vi "close_all.vi"(6 "Array of Controller Status":T1, 8 "error in (no error)":errorcluster, 9 "Hamamatsu_C9100-13.lvclass":refnum<class "Hamamatsu_C9100-13.lvclass">, 10 "HP83623A Generator Settings Array":T2, 11 "DDS Settings":T4={"Enable DDS"=TRUE, "Array of DDS Boxes"=[]} {"Array of DDS Boxes"."Array of DDS Channels (4)"."Channel Parameters"."Ref Clock Rate [kHz]" min=0.0}) -> (0 "error out":errorcluster)   [LabVIEW 2013, in "Experiment.lvclass"]
uses:
  Experiment/Experiment.lvclass
  DDS/DDS_Settings_Cluster.ctl
  DDS drivers v3/Array_of_DDS_Boxes.ctl
  DDS drivers v3/DDS_box_cluster.ctl
  DDS drivers v3/DDS_box_device_reference.ctl
  <vilib>/ni845x/ni845x.llb/ni845xControl.ctl
  DDS drivers v3/array_of_DDS_channels.ctl
  DDS drivers v3/DDS_channel.ctl
  DDS drivers v3/array_of_DDS_profiles.ctl
  DDS drivers v3/DDS_profile.ctl
  DDS drivers v3/DDS RAM mode.ctl
  GPIB/HP83623A_RF_Generator/HP83623A_array.ctl
  GPIB/HP83623A_RF_Generator/HP83623A.ctl
  Camera/Hamamatsu_C9100-13/Hamamatsu_C9100-13.lvclass
  PI_piezo/status.ctl
  GPIB/HP83623A_RF_Generator/HP83623A_RF_Generator.lvclass
  PI_piezo/PI_Piezo.lvclass
  DDS/DDS.lvclass
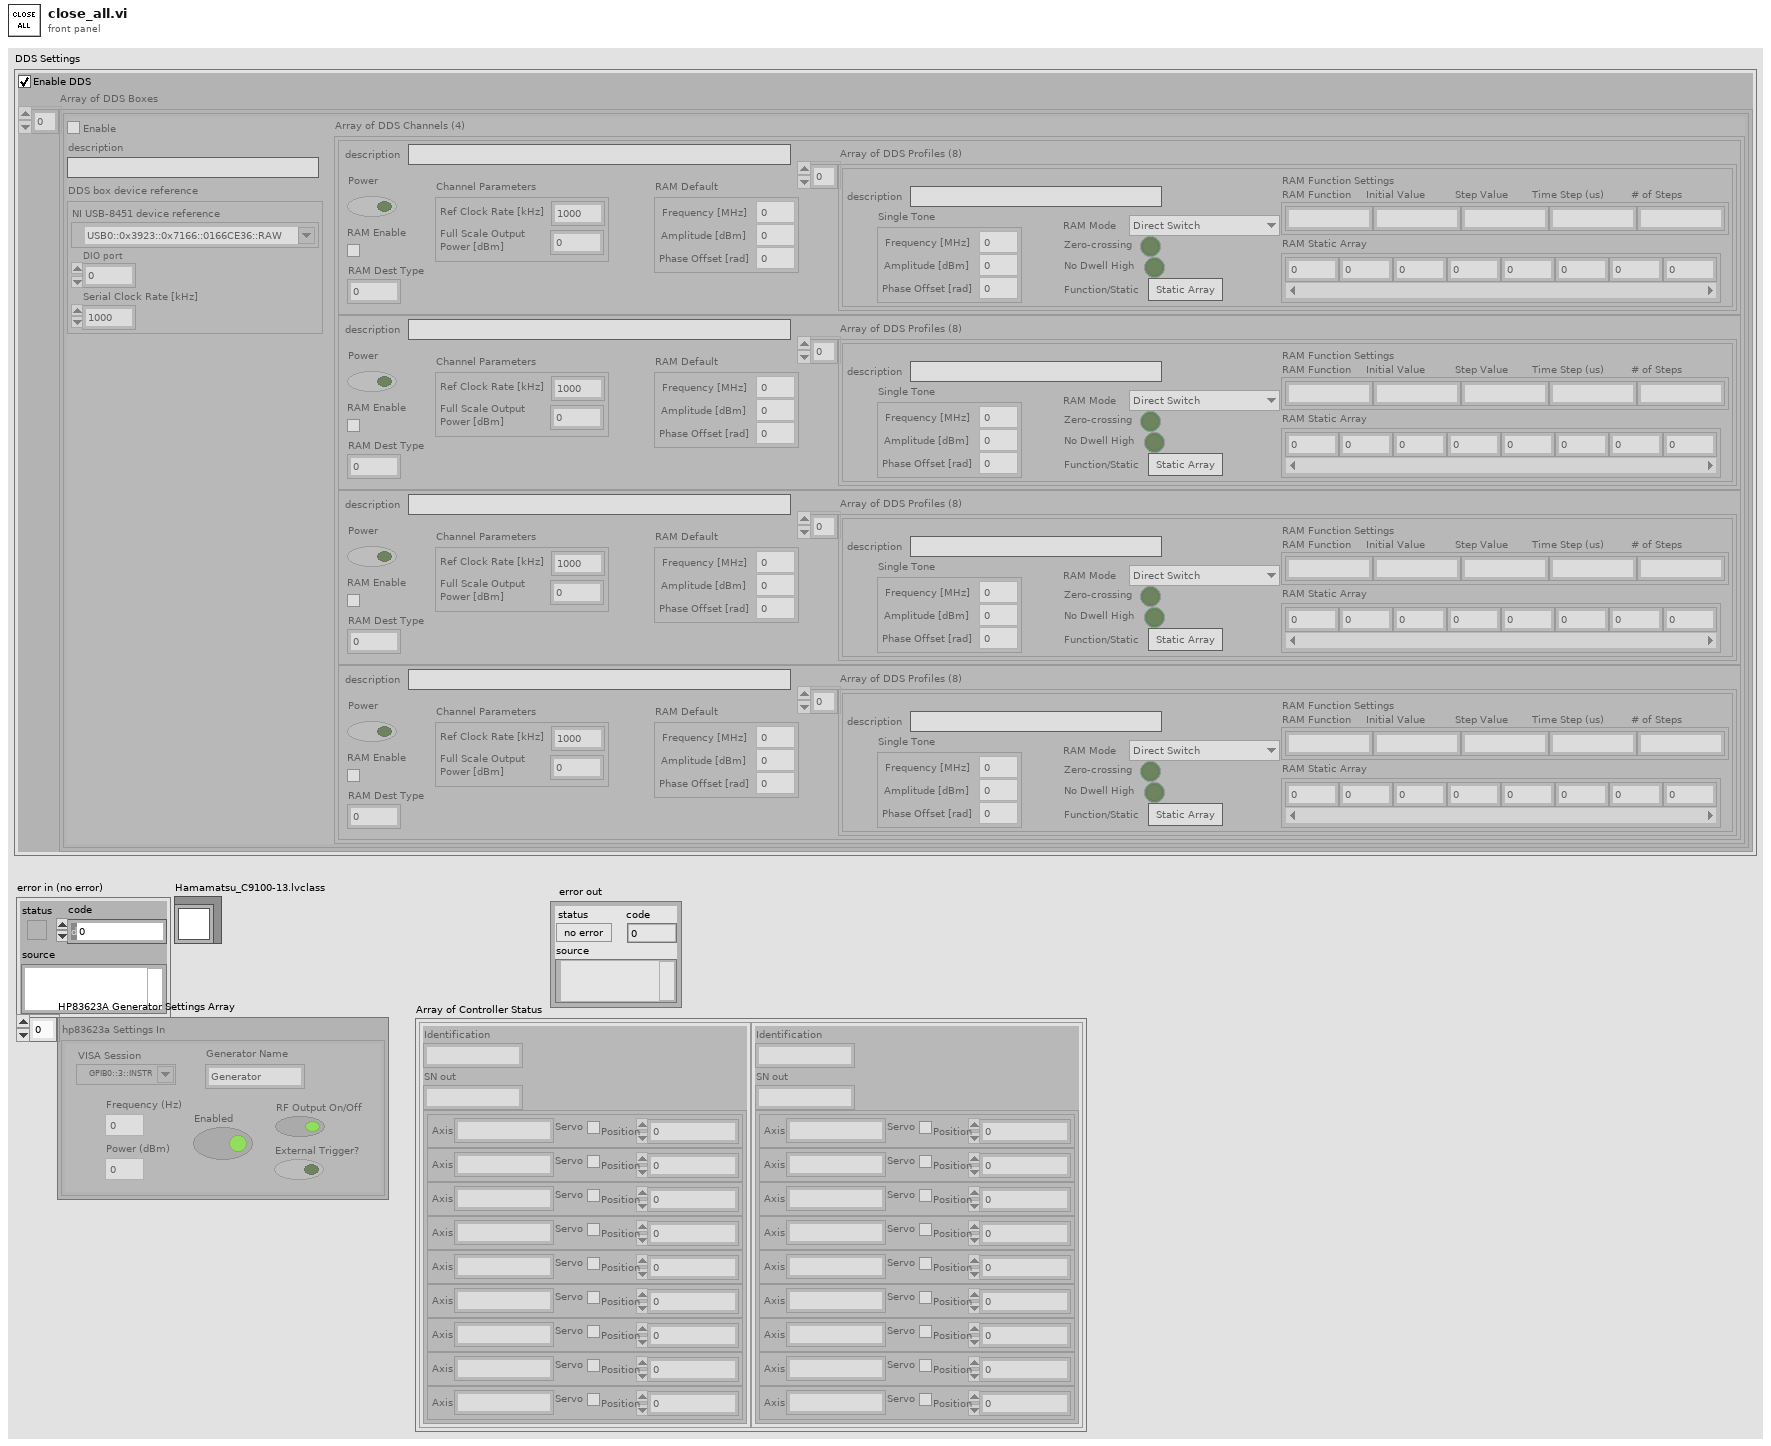
[diagram p1: front panel]
types:
  T1 = typedef "PI_Piezo.lvclass/status.ctl" = cluster{"Identification":string, "SN out":string, cluster{"Axis":string, "Servo":bool, "Position":dbl}[]}[]
  T2 = typedef "HP83623A_RF_Generator.lvclass/HP83623A_array.ctl" = T3[]
  T3 = typedef "HP83623A_RF_Generator.lvclass/HP83623A.ctl" = cluster{"Frequency (Hz)":dbl, "Power (dBm)":dbl, "Enabled":bool, "initialized":bool, "RF Output On/Off":bool, "External Trigger?":bool, "VISA Session":refnum<visa-resource-name>, "Generator Name":string}
  T4 = typedef "DDS_Settings_Cluster.ctl" = cluster{"Enable DDS":bool, "Array of DDS Boxes":T5}
  T5 = typedef "Array_of_DDS_Boxes.ctl" = T6[]
  T6 = typedef "DDS_box_cluster.ctl" = cluster{"DDS box device reference":T7, "Array of DDS Channels (4)":T9, "Enable":bool, "description":string}
  T7 = typedef "DDS_box_device_reference.ctl" = cluster{"NI USB-8451 device reference":T8, "DIO port":u8, "Serial Clock Rate [kHz]":u16}
  T8 = typedef "ni845xControl.ctl" = refnum<k21>
  T9 = typedef "DDS.lvclass/array_of_DDS_channels.ctl" = T10[]
  T10 = typedef "DDS.lvclass/DDS_channel.ctl" = cluster{"Power":bool, "Channel Parameters":cluster{"Ref Clock Rate [kHz]":dbl, "Full Scale Output\nPower [dBm]":dbl}, "RAM Enable":bool, "RAM Dest Type":u8, "RAM Default":cluster{"Frequency [MHz]":dbl, "Amplitude [dBm]":dbl, "Phase Offset [rad]":dbl}, "Array of DDS Profiles (8)":T11, "description":string}
  T11 = typedef "DDS.lvclass/array_of_DDS_profiles.ctl" = T12[]
  T12 = typedef "DDS_profile.ctl" = cluster{"Single Tone":cluster{"Frequency [MHz]":dbl, "Amplitude [dBm]":dbl, "Phase Offset [rad]":dbl}, "RAM Mode ":T13, "Zero-crossing":bool, "No Dwell High":bool, "Function/Static":bool, "RAM Function Settings":string[], "RAM Static Array":dbl[], "description":string}
  T13 = typedef "DDS RAM mode.ctl" = enum16{"Direct Switch", "Ramp Up", "Bidirectional Ramp", "Continuous Bidirectional Ramp", "Continuous Recirculate", "Direct Switch 2", "Direct Switch 3", "Direct Switch 4"}
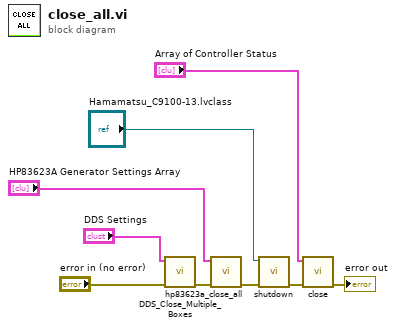
[diagram p0: block diagram]
diagram:
  n1 = call "DDS_Close_Multiple_Boxes.vi"("error in (no error)"="error in (no error)", "DDS Settings"="DDS Settings") -> ("error out"=w8:errorcluster)  [unwired: 9 in]
  n2 = call "hp83623a_close_all.vi"("error in"=w8, "HP83623A Generator Settings Array"="HP83623A Generator Settings Array") -> ("error out"=w6:errorcluster)  [unwired: 9 in]
  n3 = call-dynamic "shutdown.vi"("error in (no error)"=w6, "Hamamatsu_C9100-13 in"="Hamamatsu_C9100-13.lvclass") -> ("error out"=w5:errorcluster)  [unwired: 8 in, 1 out]
  n4 = call "close.vi"("error in"=w5, "Array of Controller Status"="Array of Controller Status") -> ("error out"=→"error out":errorcluster)  [unwired: 9 in]
